vi "SetSimbolToT.vi"(10 "index":i32, 11 "ProcessList":refnum<vi>) -> ()   [LabVIEW 2019]
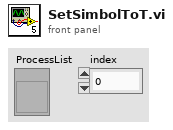
[diagram p1: front panel]
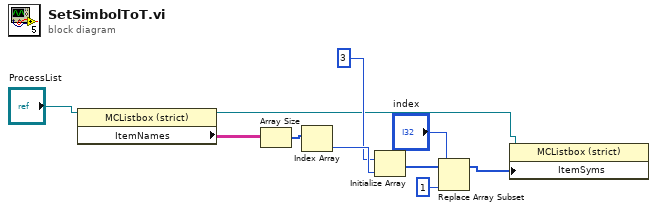
[diagram p0: block diagram]
diagram:
  n1 = property class="MCListbox (strict)"(reference="ProcessList") -> (reference out=w4:refnum<vi>, "ItemNames"=w9:string[][])  [unwired: 1 in, 1 out]
  n2 = Array Size(array=w9) -> (size(s)=w8:i32[])
  n3 = Index Array(array=w8) -> (element=w7:i32)  [unwired: 1 in]
  n4 = Initialize Array(3 ("element"), w7) -> (w5:i32[])
  n5 = Replace Array Subset(array=w5, new element=1 ("new element/subarray"), index="index") -> (w3:i32[])
  n6 = property class="MCListbox (strict)"(reference=w4, "ItemSyms"=w3) -> ()  [unwired: 1 in, 2 out]
